vi "getLaguerreBasis.vi"(8 "error in (no error)":errorcluster, 11 "LaguerreDeconClass in":refnum<class "LaguerreDeconEngineClass.lvclass">) -> (0 "error out":errorcluster, 2 "laguerreBasis":dbl[][](array[numeric]), 3 "LaguerreDeconClass out":refnum<class "LaguerreDeconEngineClass.lvclass">)   [LabVIEW 2024, in "LaguerreDeconEngineClass.lvclass"]
uses:
  LaguerreDeconEngineClass.lvclass
  LaguerreDeconEngineClass.lvclass/LaguerreDeconEngineClass.ctl
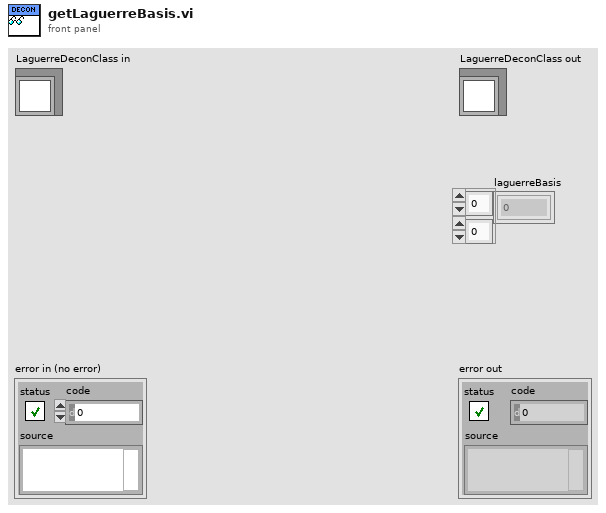
[diagram p1: front panel]
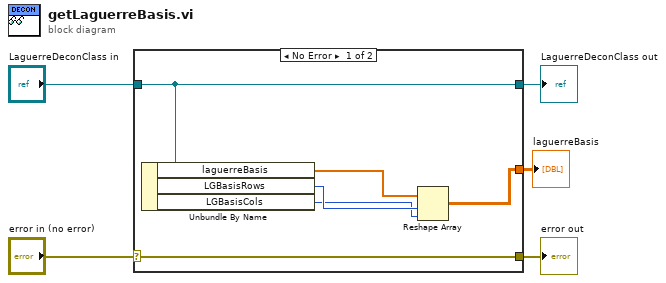
[diagram p0: block diagram]
diagram:
  n1 = case shown="No Error" "error in (no error)" {
    selector: "error in (no error)" -> [w11 w12]
    tunnel: [w11 w12] -> w4
    tunnel: [w10 w13] -> w2
    tunnel: "LaguerreDeconClass in" -> [w10 w13]
    tunnel: [w6 _] -> w1
    frame No Error {
      n2 = Unbundle By Name(w10) -> ("laguerreBasis"=w9:dbl[], "LGBasisRows"=w8:u64, "LGBasisCols"=w7:u64)
      n3 = Reshape Array(w9, w8, w7) -> (w6:dbl[][])
    }
    frame Error {
    }
  }
  "error out" <- w4
  "LaguerreDeconClass out" <- w2
  "laguerreBasis" <- w1
